vi "Async Consumer Launcher.vi"(8 "error in (no error)":errorcluster, 11 "Consumers":refnum<class "Abstract Consumer.lvclass">[](array[class])) -> (0 "error out":errorcluster)   [LabVIEW 2027, in "Multi Consumer Test Case.lvclass"]
uses:
  Multi Consumer Test Case.lvclass
  Consumer/Abstract Consumer/Abstract Consumer.lvclass
  Execute Message Async.vi
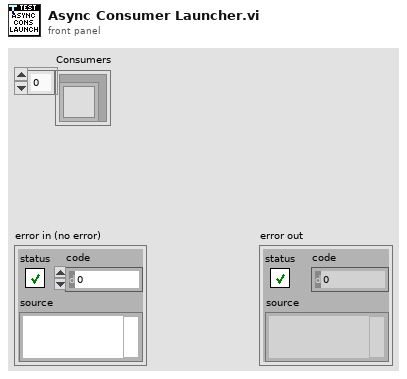
[diagram p1: front panel]
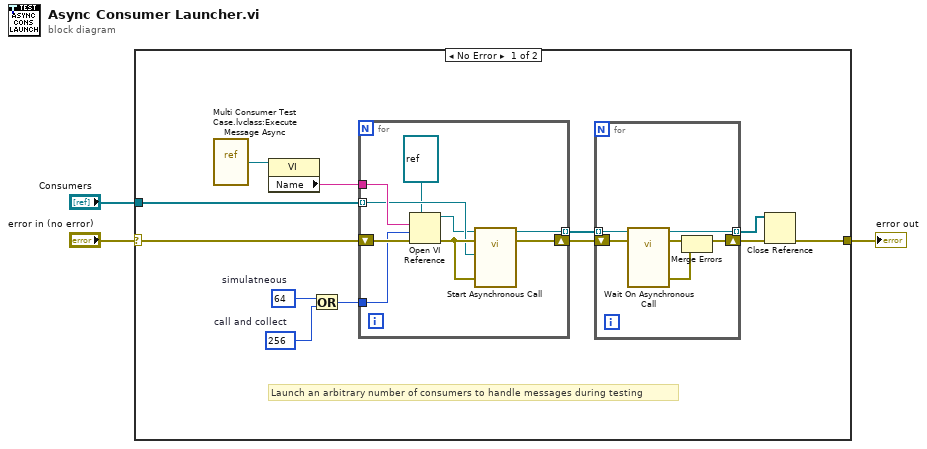
[diagram p0: block diagram]
diagram:
  n1 = case shown="No Error" "error in (no error)" {
    selector: "error in (no error)" -> [w4 w31]
    tunnel: "Consumers" -> [w6 _]
    tunnel: [w5 w31] -> w2
    frame No Error {
      w9 = 64  # simulatneous
      w8 = 256  # call and collect
      # "Launch an arbitrary number of consumers to handle messages during testing"
      n2 = vi-ref "Multi Consumer Test Case.lvclass:Execute Message Async.vi"() -> (w15:refnum<vi>)
      n3 = property class="VI"(reference=w15) -> ("Name"=w14:string)  [unwired: 1 in, 2 out]
      n4 = Or(x=w9, y=w8) -> (x .or. y?=w7:i32)
      n5 = for {
        tunnel: w6 -> [w26] mode=indexing
        tunnel: w14 -> [w30]
        shift-right: [w25] -> w13
        shift-left: w4 -> [w29]
        tunnel: w7 -> [w28]
        tunnel: [w24] -> w12 mode=indexing
        n6 = Open VI Reference(type specifier VI Refnum (for type only)=refnum<vi> refnum, vi path=w30, options=w28, error in (no error)=w29) -> (vi reference=w22:refnum<vi>, error out=w27:errorcluster)  [unwired: 2 in]
        n7 = call-by-ref "Start Asynchronous Call"(reference=w22, error in=w27, 8:"error in (no error)"=w27, "Consumer"=w26) -> (reference out=w24:refnum<vi>, error out=w25:errorcluster)  [unwired: 9 in, 1 out]
      }
      n8 = for {
        shift-right: [w18] -> w11
        shift-left: w13 -> [w20]
        tunnel: w12 -> [w21] mode=indexing
        tunnel: [w17] -> w10 mode=indexing
        n9 = call-by-ref "Wait On Asynchronous Call"(reference=w21, error in=w20) -> (reference out=w17:refnum<vi>, error out=w16:errorcluster, 0:"error out"=w19:errorcluster)  [unwired: 11 in]
        n10 = Merge Errors(w16, w19) -> (w18:errorcluster)
      }
      n11 = Close Reference(reference=w10, error in (no error)=w11) -> (error out=w5:errorcluster)
    }
    frame Error {
    }
  }
  "error out" <- w2
